vi "Experiment 1.vi"() -> ()   [LabVIEW 2026]
panel:
  out "Execution Time (seconds)":dbl format="%.6f"
  out "Output":dbl[](array[numeric]) format="%.3f"
  # "Experiment 1"
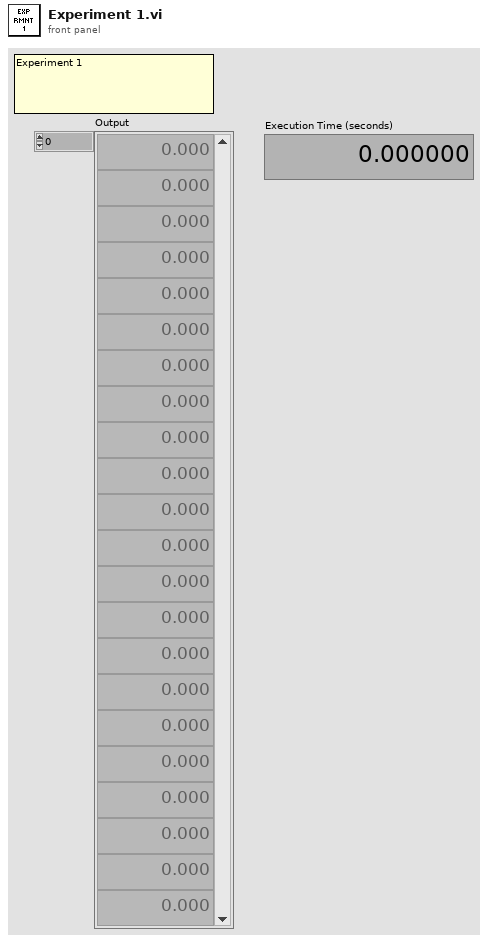
[diagram p1: front panel]
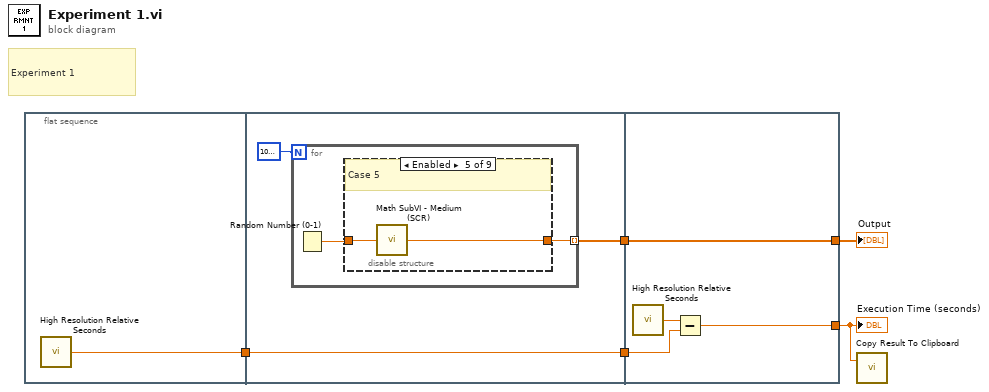
[diagram p0: block diagram]
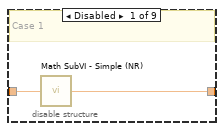
[diagram p2: hidden frame]
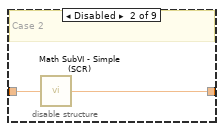
[diagram p3: hidden frame]
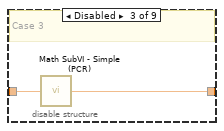
[diagram p4: hidden frame]
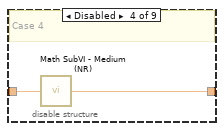
[diagram p5: hidden frame]
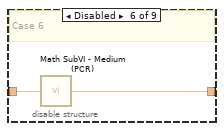
[diagram p6: hidden frame]
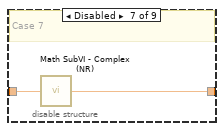
[diagram p7: hidden frame]
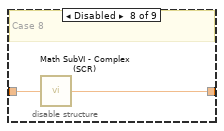
[diagram p8: hidden frame]
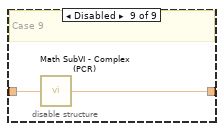
[diagram p9: hidden frame]
diagram:
  # "Experiment 1"
  n1 = flat-sequence {
    tunnel: [w6] -> w5
    tunnel: w5 -> [w9]
    tunnel: [w9] -> w4
    tunnel: [w7] -> w3
    tunnel: w4 -> [w32]
    tunnel: w3 -> [w31]
    tunnel: [w31] -> w2
    tunnel: [w30] -> w1
    frame #0 {
      n2 = call <vilib>:"High Resolution Relative Seconds.vi"() -> ("relative seconds"=w6:dbl)
    }
    frame #1 {
      n3 = for {
        N: 1000000 -> [_]
        tunnel: [w11] -> w7 mode=indexing
        n4 = Random Number (0-1)() -> (number: 0 to 1=w10:dbl)
        n5 = disable-structure shown="Enabled" {
          disable-tunnel: [w13 w15 w17 w19 w21 w23 w25 w27 w29] -> w11
          disable-tunnel: w10 -> [w12 w14 w16 w18 w20 w22 w24 w26 w28]
          frame Disabled {
            # "Case 1"
            n6 = call "Math SubVI - Simple (NR).vi"("Input"=w12) -> ("Output"=w13:dbl)
          }
          frame Disabled {
            # "Case 2"
            n7 = call "Math SubVI - Simple (SCR).vi"("Input"=w14) -> ("Output"=w15:dbl)
          }
          frame Disabled {
            # "Case 3"
            n8 = call "Math SubVI - Simple (PCR).vi"("Input"=w16) -> ("Output"=w17:dbl)
          }
          frame Disabled {
            # "Case 4"
            n9 = call "Math SubVI - Medium (NR).vi"("Input"=w18) -> ("Output"=w19:dbl)
          }
          frame Enabled {
            # "Case 5"
            n10 = call "Math SubVI - Medium (SCR).vi"("Input"=w20) -> ("Output"=w21:dbl)
          }
          frame Disabled {
            # "Case 6"
            n11 = call "Math SubVI - Medium (PCR).vi"("Input"=w22) -> ("Output"=w23:dbl)
          }
          frame Disabled {
            # "Case 7"
            n12 = call "Math SubVI - Complex (NR).vi"("Input"=w24) -> ("Output"=w25:dbl)
          }
          frame Disabled {
            # "Case 8"
            n13 = call "Math SubVI - Complex (SCR).vi"("Input"=w26) -> ("Output"=w27:dbl)
          }
          frame Disabled {
            # "Case 9"
            n14 = call "Math SubVI - Complex (PCR).vi"("Input"=w28) -> ("Output"=w29:dbl)
          }
        }
      }
    }
    frame #2 {
      n15 = call <vilib>:"High Resolution Relative Seconds.vi"() -> ("relative seconds"=w33:dbl)
      n16 = Subtract(x=w33, y=w32) -> (x-y=w30:dbl)
    }
  }
  n17 = call "Copy Result To Clipboard.vi"("Input"=w1) -> ()  [unwired: 1 in]
  "Output" <- w2
  "Execution Time (seconds)" <- w1
